vi "CreateVirtualChannels.vi"(8 "error in (no error)":errorcluster, 9 "data in":T1, 11 "virtual channel config in":T5) -> (0 "error out":errorcluster, 1 "data out":T1, 3 "virtual channel config out":T5)   [LabVIEW 2017, in "CmsVirtualChannel.lvlib"]
uses:
  <vilib>/addons/InsightCM/Devices/Shared/Cms/CmsVirtualChannel/CmsVirtualChannel.lvlib
  <vilib>/addons/InsightCM/Devices/Shared/Cms/CmsVirtualChannel/controls/Config.ctl
  <vilib>/addons/InsightCM/Devices/Shared/Cms/CmsVirtualChannel/controls/VirtualChannelGroup.ctl
  <vilib>/addons/InsightCM/Devices/Shared/Cms/CmsVirtualChannel/controls/VirtualChannel.ctl
  <vilib>/addons/InsightCM/Devices/Shared/Common/DataFlow/controls/Data.ctl
  <vilib>/addons/InsightCM/Utilities/DataAccessors/controls/wfmSGL_DVR.ctl
  <vilib>/addons/PointValueMap/controls/PointMap.ctl
  <vilib>/addons/InsightCM/Devices/Shared/Common/DataFlow/controls/Type.ctl
  <vilib>/addons/PointValueMap/PointValueMap.lvlib
  <vilib>/addons/InsightCM/Devices/Shared/Common/DataFlow/DataFlow.lvlib
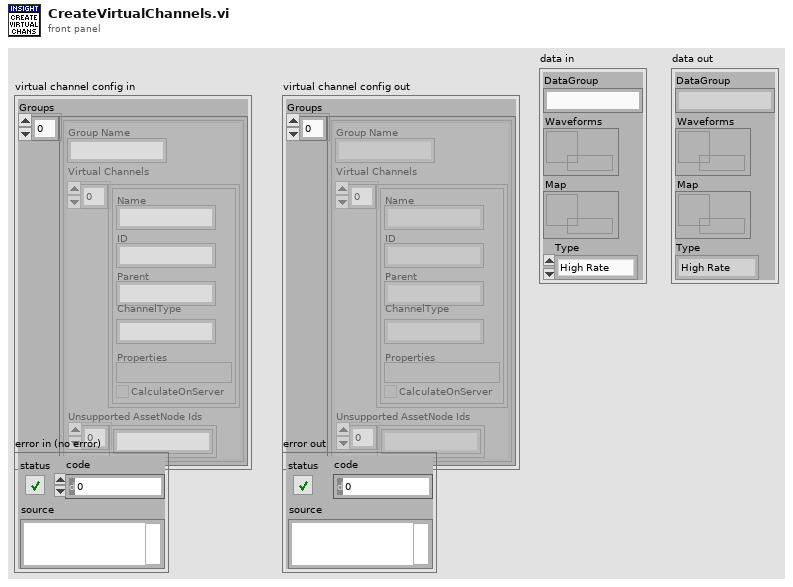
[diagram p1: front panel]
types:
  T1 = typedef "DataFlow.lvlib/Data.ctl" = cluster{"DataGroup":string, "Waveforms":T2, "Map":T3, "Type":T4}
  T2 = typedef "wfmSGL_DVR.ctl" = refnum<data-value>
  T3 = typedef "PointValueMap.lvlib/PointMap.ctl" = refnum<data-value>
  T4 = typedef "DataFlow.lvlib/Type.ctl" = enum16{"High Rate", "Low Rate", "Burst Mode"}
  T5 = typedef "CmsVirtualChannel.lvlib/Config.ctl" = cluster{"Groups":T6[]}
  T6 = typedef "CmsVirtualChannel.lvlib/VirtualChannelGroup.ctl" = cluster{"Group Name":string, "Virtual Channels":T7[], "Unsupported AssetNode Ids":string[]}
  T7 = typedef "CmsVirtualChannel.lvlib/VirtualChannel.ctl" = cluster{"Name":string, "ID":string, "Parent":string, "ChannelType":string, "Properties":variant, "CalculateOnServer":bool}
  T8 = typedef "AnalysisHelper.lvlib/PulsePositions.ctl" = cluster{"Name":string, "Pulse Position Data":dbl[], "Pulses Per Rev":i32}
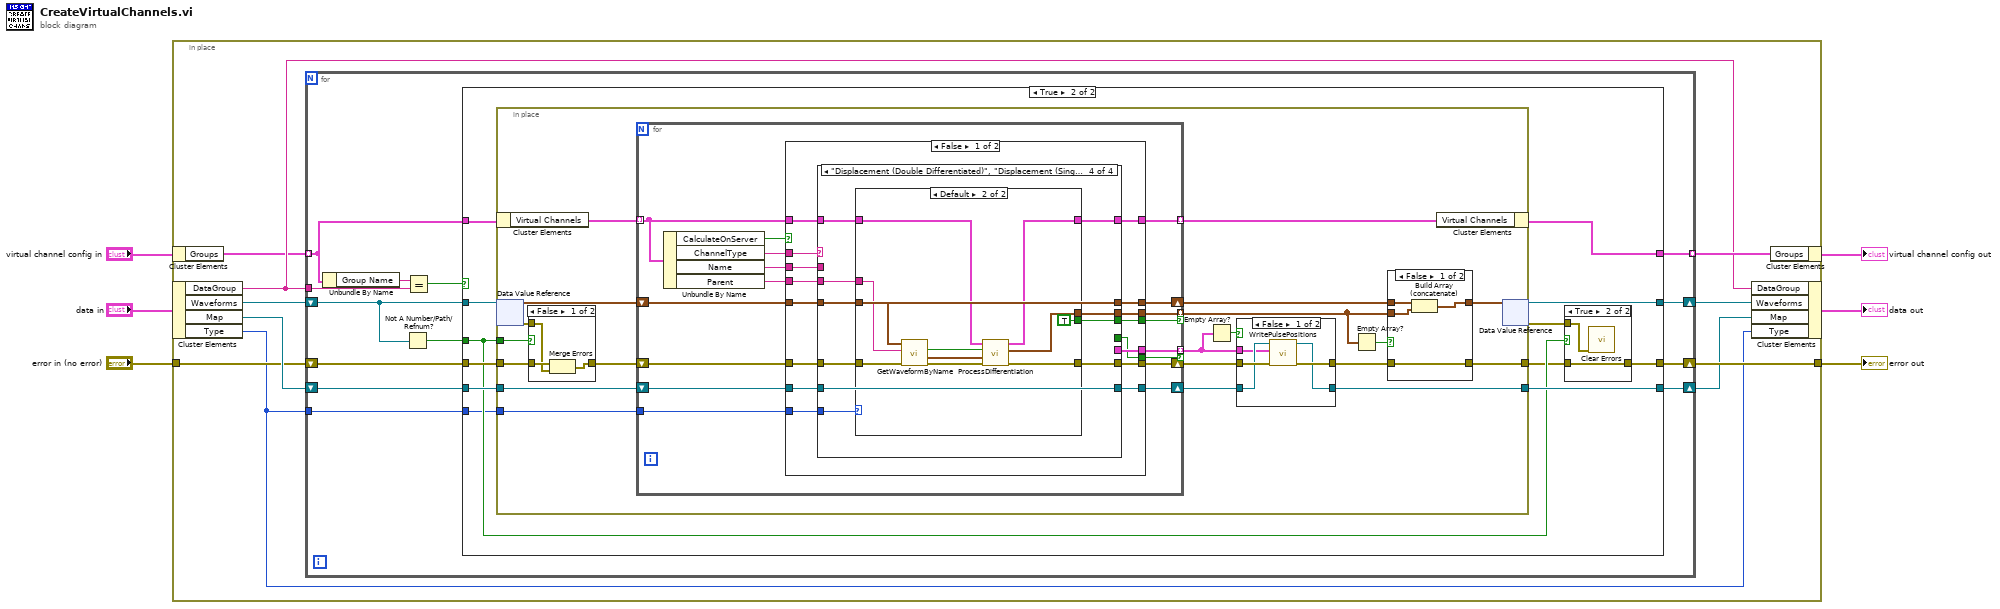
[diagram p0: block diagram]
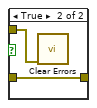
[diagram p4: hidden frame]
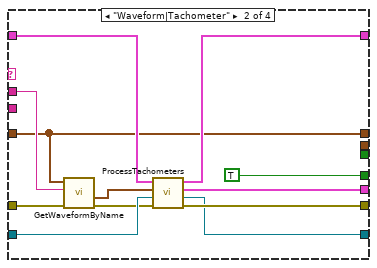
[diagram p7: hidden frame]
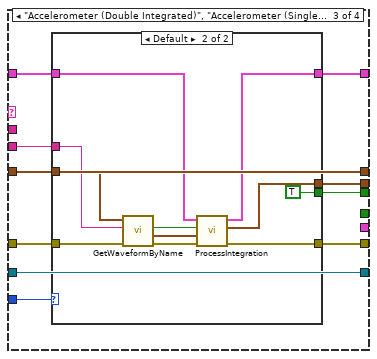
[diagram p8: hidden frame]
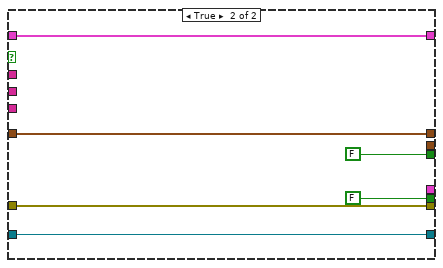
[diagram p11: hidden frame]
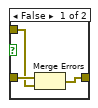
[diagram p12: hidden frame]
diagram:
  n1 = in-place {
    in-place-border: "error in (no error)" -> [w13]
    in-place-border: [w11] -> w1
    n2 = in-place-cluster #1("virtual channel config in") -> ("Groups"=w10:T6[])
    n3 = in-place-cluster #2("data in") -> ("DataGroup"=w12:string, "Waveforms"=w15:T2, "Map"=w14:T3, "Type"=w9:T4)
    n4 = for {
      tunnel: w10 -> [w27] mode=indexing
      tunnel: w12 -> [w28]
      tunnel: [w21] -> w16 mode=indexing
      shift-right: [w20] -> w11
      shift-left: w13 -> [w25]
      tunnel: w9 -> [w19]
      shift-right: [w18] -> w8
      shift-left: w15 -> [w24]
      shift-right: [w17] -> w7
      shift-left: w14 -> [w26]
      n5 = Unbundle By Name(w27) -> ("Group Name"=w29:string)
      n6 = Not A Number/Path/Refnum?(number/path/refnum=w24) -> (NaN/Path/Refnum?=w22:bool)
      n7 = Equal?(x=w29, y=w28) -> (x = y?=w23:bool)
      n8 = case shown="True" w23 {
        tunnel: w27 -> [w33 w43]
        tunnel: w24 -> [w31 w41]
        tunnel: w26 -> [w30 w45]
        tunnel: w25 -> [w32 w44]
        tunnel: [w33 w42] -> w21
        tunnel: [w32 w35] -> w20
        tunnel: [w30 w40] -> w17
        tunnel: [w31 w39] -> w18
        tunnel: w22 -> [_ w37]
        tunnel: w19 -> [_ w34]
        frame False {
        }
        frame True {
          n9 = in-place {
            in-place-border: w45 -> [w65]
            in-place-border: w44 -> [w56]
            in-place-border: [w54] -> w36
            in-place-border: [w52] -> w40
            in-place-border: w37 -> [w58]
            in-place-border: w34 -> [w48]
            n10 = in-place-cluster #3(w43) -> ("Virtual Channels"=w64:T7[])
            n11 = in-place-dvr #4(w41) -> (w62:waveform(sgl)[], w57:errorcluster)
            n12 = case shown="False" w58 {
              tunnel: w57 -> [w72 w76]
              tunnel: w56 -> [w73 w75]
              tunnel: [w74 w75] -> w55
              frame False {
                n13 = Merge Errors(w73, w72) -> (w74:errorcluster)
              }
              frame True {
                n14 = call <vilib>:"Clear Errors.vi"("error in (no error)"=w76) -> ()  [unwired: 5 in, 2 out]
              }
            }
            n15 = for {
              tunnel: w64 -> [w96] mode=indexing
              tunnel: [w97] -> w63 mode=indexing
              shift-right: [w94] -> w61
              shift-left: w55 -> [w100]
              tunnel: [w93] -> w59 mode=indexing if=w92
              tunnel: [w91] -> w51 mode=indexing if=w90
              tunnel: w48 -> [w88]
              shift-right: [w85] -> w47
              shift-left: w65 -> [w95]
              shift-right: [w84] -> w46
              shift-left: w62 -> [w99]
              n16 = Unbundle By Name(w96) -> ("CalculateOnServer"=w89:bool, "ChannelType"=w98:string, "Name"=w87:string, "Parent"=w86:string)
              n17 = case shown="False" w89 {
                tunnel: w100 -> [w116 w180]
                tunnel: w99 -> [w115 w183]
                tunnel: w98 -> [w114 _]
                tunnel: [w113 w184] -> w97
                tunnel: w96 -> [w112 w184]
                tunnel: w95 -> [w111 w181]
                tunnel: [w110 w181] -> w85
                tunnel: [w109 w180] -> w94
                tunnel: [w108 _] -> w93
                tunnel: [w107 FALSE] -> w92
                tunnel: [w106 _] -> w91
                tunnel: [w105 FALSE] -> w90
                tunnel: [w104 w183] -> w84
                tunnel: w88 -> [w103 _]
                tunnel: w87 -> [w102 _]
                tunnel: w86 -> [w101 _]
                frame False {
                  n18 = case shown="\"Displacement (Double Differentiated)\", \"Displacement (Single Differentiated)\", \"Velocity (Single Differentiated)\"" w114 {
                    tunnel: w116 -> [w119 w122 w141 w164]
                    tunnel: w115 -> [w118 w124 w137 w160]
                    tunnel: [w119 w129 w140 w163] -> w109
                    tunnel: [w120 w131 w139 w162] -> w113
                    tunnel: w112 -> [w120 w132 w142 w165]
                    tunnel: [w118 w124 w137 w160] -> w104
                    tunnel: [w117 w128 w138 w161] -> w110
                    tunnel: w111 -> [w117 w130 w138 w161]
                    tunnel: [_ w127 _ _] -> w108
                    tunnel: [_ TRUE _ _] -> w107
                    tunnel: [_ _ w136 w159] -> w106
                    tunnel: [_ _ w135 w158] -> w105
                    tunnel: w103 -> [_ _ w134 w157]
                    tunnel: w102 -> [_ w125 _ _]
                    tunnel: w101 -> [_ _ w133 w156]
                    frame Default {
                    }
                    frame "Waveform|Tachometer" {
                      n19 = call <vilib>:"GetWaveformByName.vi"("error in (no error)"=w122, "Channel Name"=w125, "Acq Waveforms"=w124) -> ("error out"=w121:errorcluster, "Waveform"=w123:waveform(sgl))  [unwired: 5 in, 2 out]
                      n20 = call <vilib>:"ProcessTachometers.vi"("error in (no error)"=w121, "map"=w130, "Waveform"=w123, "virtual channel in"=w132) -> ("error out"=w129:errorcluster, "map out"=w128:T3, "pulse positions"=w127:T8, "virtual channel out"=w131:T7)  [unwired: 4 in]
                    }
                    frame "Accelerometer (Double Integrated)", "Accelerometer (Single Integrated)", "Velocity (Single Integrated)" {
                      n21 = case shown="Default" w134 {
                        tunnel: w142 -> [w144 w155]
                        tunnel: w141 -> [w143 w148]
                        tunnel: [w143 w154] -> w140
                        tunnel: [w144 w153] -> w139
                        tunnel: w137 -> [_ w149]
                        tunnel: [_ w152] -> w136
                        tunnel: [_ TRUE] -> w135
                        tunnel: w133 -> [_ w150]
                        frame "Burst Mode" {
                        }
                        frame Default {
                          n22 = call <vilib>:"GetWaveformByName.vi"("error in (no error)"=w148, "Channel Name"=w150, "Acq Waveforms"=w149) -> ("error out"=w147:errorcluster, "Waveform"=w145:waveform(sgl), "Found?"=w146:bool)  [unwired: 5 in, 1 out]
                          n23 = call <vilib>:"ProcessIntegration.vi"("error in (no error)"=w147, "parent waveform"=w145, "parent found"=w146, "virtual channel"=w155) -> ("error out"=w154:errorcluster, "integrated waveform"=w152:waveform(sgl), "virtual channel out"=w153:T7)  [unwired: 5 in]
                        }
                      }
                    }
                    frame "Displacement (Double Differentiated)", "Displacement (Single Differentiated)", "Velocity (Single Differentiated)" {
                      n24 = case shown="Default" w157 {
                        tunnel: w165 -> [w167 w178]
                        tunnel: w164 -> [w166 w173]
                        tunnel: [w166 w177] -> w163
                        tunnel: [w167 w176] -> w162
                        tunnel: w160 -> [_ w171]
                        tunnel: [_ w175] -> w159
                        tunnel: [_ TRUE] -> w158
                        tunnel: w156 -> [_ w170]
                        frame "Burst Mode" {
                        }
                        frame Default {
                          n25 = call <vilib>:"GetWaveformByName.vi"("error in (no error)"=w173, "Channel Name"=w170, "Acq Waveforms"=w171) -> ("error out"=w172:errorcluster, "Waveform"=w168:waveform(sgl), "Found?"=w169:bool)  [unwired: 5 in, 1 out]
                          n26 = call <vilib>:"ProcessDifferentiation.vi"("error in (no error)"=w172, "parent waveform"=w168, "parent found"=w169, "virtual channel"=w178) -> ("error out"=w177:errorcluster, "differentiated channel"=w175:waveform(sgl), "virtual channel out"=w176:T7)  [unwired: 5 in]
                        }
                      }
                    }
                  }
                }
                frame True {
                }
              }
            }
            n27 = Empty Array?(array=w59) -> (empty?=w60:bool)
            n28 = case shown="False" w60 {
              tunnel: w61 -> [w81 w83]
              tunnel: [w80 w83] -> w53
              tunnel: w47 -> [w79 w82]
              tunnel: [w78 w82] -> w52
              tunnel: w59 -> [w77 _]
              frame False {
                n29 = call <vilib>:"WritePulsePositions.vi"("error in (no error)"=w81, "pulse positions array"=w77, "map in"=w79) -> ("error out"=w80:errorcluster, "map out"=w78:T3)  [unwired: 7 in]
              }
              frame True {
              }
            }
            n30 = Empty Array?(array=w51) -> (empty?=w49:bool)
            n31 = case shown="False" w49 {
              tunnel: [w66 w70] -> w54
              tunnel: w53 -> [w66 w70]
              tunnel: w51 -> [w67 _]
              tunnel: w46 -> [w69 w71]
              tunnel: [w68 w71] -> w50
              frame False {
                n32 = Build Array (concatenate)(w69, w67) -> (w68:waveform(sgl)[])
              }
              frame True {
              }
            }
            n33 = in-place-cluster #3("Virtual Channels"=w63) -> (w42:T6)
            n34 = in-place-dvr #4(w50) -> (w39:T2, w38:errorcluster)
          }
          n35 = case shown="True" w37 {
            tunnel: w38 -> [w185 w189]
            tunnel: w36 -> [w186 w188]
            tunnel: [w187 w188] -> w35
            frame False {
              n36 = Merge Errors(w186, w185) -> (w187:errorcluster)
            }
            frame True {
              n37 = call <vilib>:"Clear Errors.vi"("error in (no error)"=w189) -> ()  [unwired: 5 in, 2 out]
            }
          }
        }
      }
    }
    n38 = in-place-cluster #2("DataGroup"=w12, "Waveforms"=w8, "Map"=w7, "Type"=w9) -> (→"data out":T1)
    n39 = in-place-cluster #1("Groups"=w16) -> (→"virtual channel config out":T5)
  }
  "error out" <- w1
